vi "IMU.vi"(8 "error in (no error)":errorcluster, 10 "Acc/Gyro  address":u8, 11 "I2C Ref":T1) -> (3 "error out":errorcluster, 5 "IMU Acc":cluster{dbl, dbl, dbl}(graph), 6 "IMU Gyro":cluster{dbl, dbl, dbl}(graph))   [LabVIEW 2019]
uses:
  <vilib>/myRIO/Instrument Drivers/Onboard IO/I2C/typedefs/I2C Reference.ctl
  <vilib>/myRIO/Common/Instrument Driver Framework/Utilities/typedefs/myRIO Generic Hardware Reference.ctl
  <vilib>/myRIO/Common/Instrument Driver Framework/Utilities/typedefs/Hardware Version Enum.ctl
  <vilib>/myRIO/Common/Instrument Driver Framework/Utilities/typedefs/myRIO v1.0 Reference.ctl
  <vilib>/myRIO/Common/Instrument Driver Framework/Utilities/typedefs/Generic FPGA Reference.ctl
  <vilib>/myRIO/Common/Instrument Driver Framework/myRIO v1.0/I2C/typedefs/I2C Channels Enum.ctl
  <vilib>/myRIO/Instrument Drivers/Onboard IO/I2C/typedefs/I2C Configuration.ctl
  <vilib>/myRIO/Instrument Drivers/Onboard IO/I2C/typedefs/I2C Transfer Rate.ctl
  <vilib>/Utility/error.llb/Error Cluster From Error Code.vi
  <vilib>/myRIO/Common/Instrument Driver Framework/myRIO v1.0/I2C/vis/myRIO v1.0 Write I2C.vi
  <vilib>/myRIO/Common/Instrument Driver Framework/myRIO v1.0/I2C/vis/myRIO v1.0 Read I2C.vi
  <vilib>/myRIO/Instrument Drivers/Onboard IO/I2C/I2C.lvlib
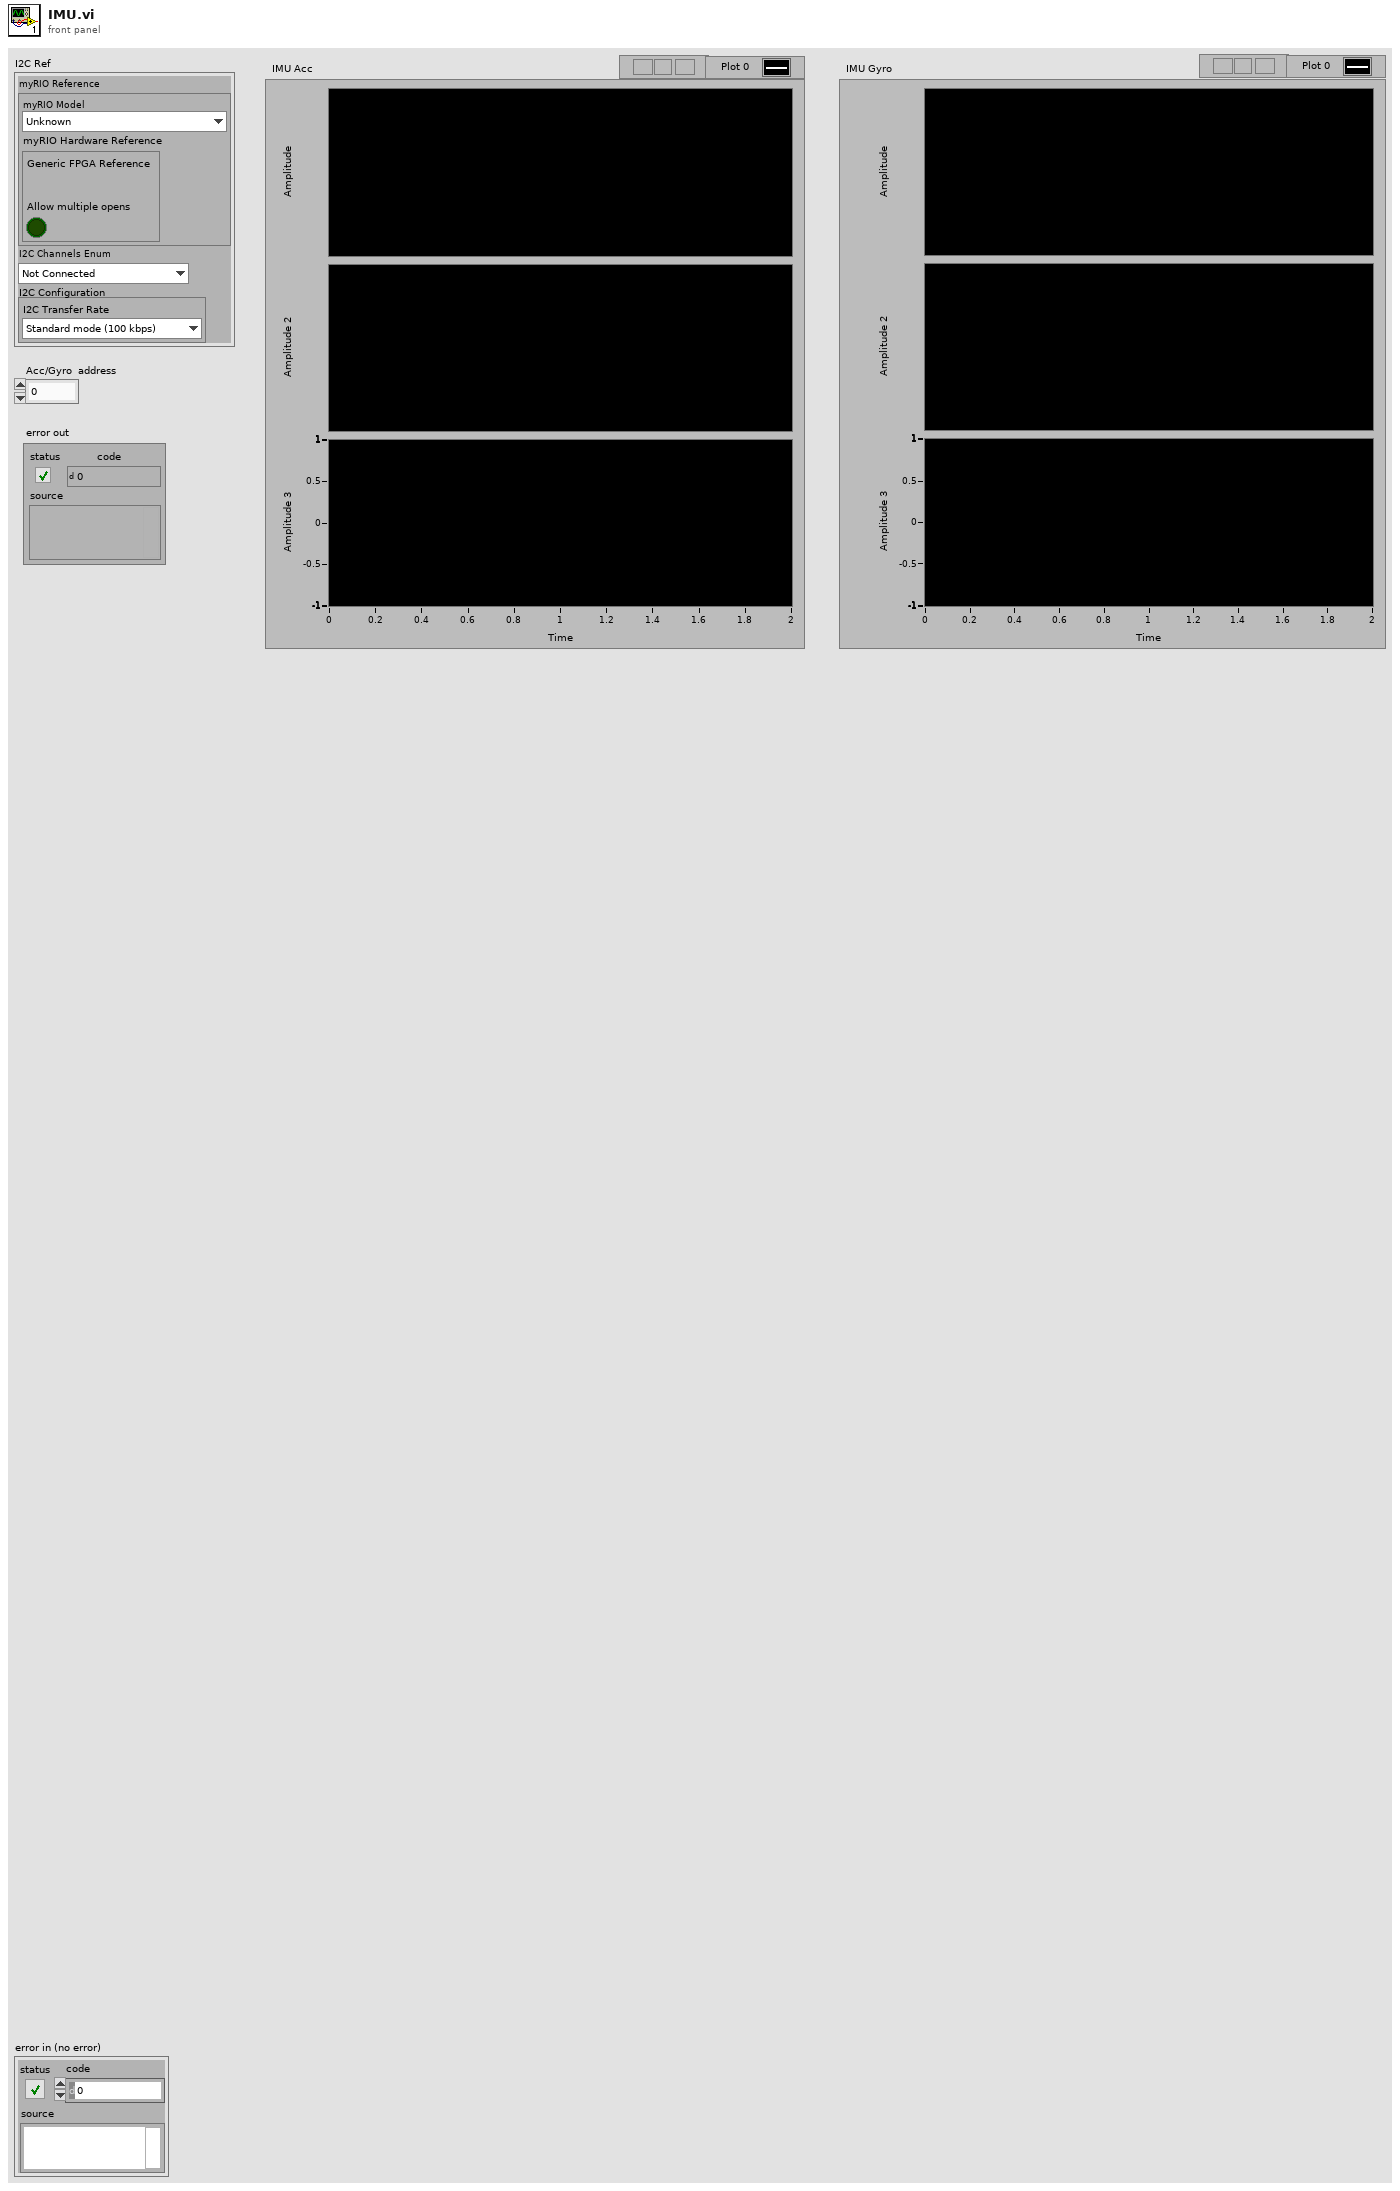
[diagram p1: front panel]
types:
  T1 = typedef "I2C.lvlib/I2C Reference.ctl" = cluster{"myRIO Reference":T2, "I2C Channels Enum":T6, "I2C Configuration":T7}
  T2 = typedef "myRIO Generic Hardware Reference.ctl" = cluster{"myRIO Model":T3, "myRIO Hardware Reference":T4}
  T3 = typedef "Hardware Version Enum.ctl" = enum16{"Unknown", "myRIO-1900", "myRIO-1950", "roboRIO", "NI ELVIS RIO CM", "ELVIS III"}
  T4 = typedef "myRIO v1.0 Reference.ctl" = cluster{"Generic FPGA Reference":T5, "Allow multiple opens":bool}
  T5 = typedef "Generic FPGA Reference.ctl" = refnum<k20>
  T6 = typedef "I2C Channels Enum.ctl" = enum16{"Not Connected", "A/I2C", "B/I2C", "I2C/I2C"}
  T7 = typedef "I2C.lvlib/I2C Configuration.ctl" = cluster{"I2C Transfer Rate":T8}
  T8 = typedef "I2C.lvlib/I2C Transfer Rate.ctl" = enum16{"Standard mode (100 kbps)", "Fast mode (400 kbps)"}
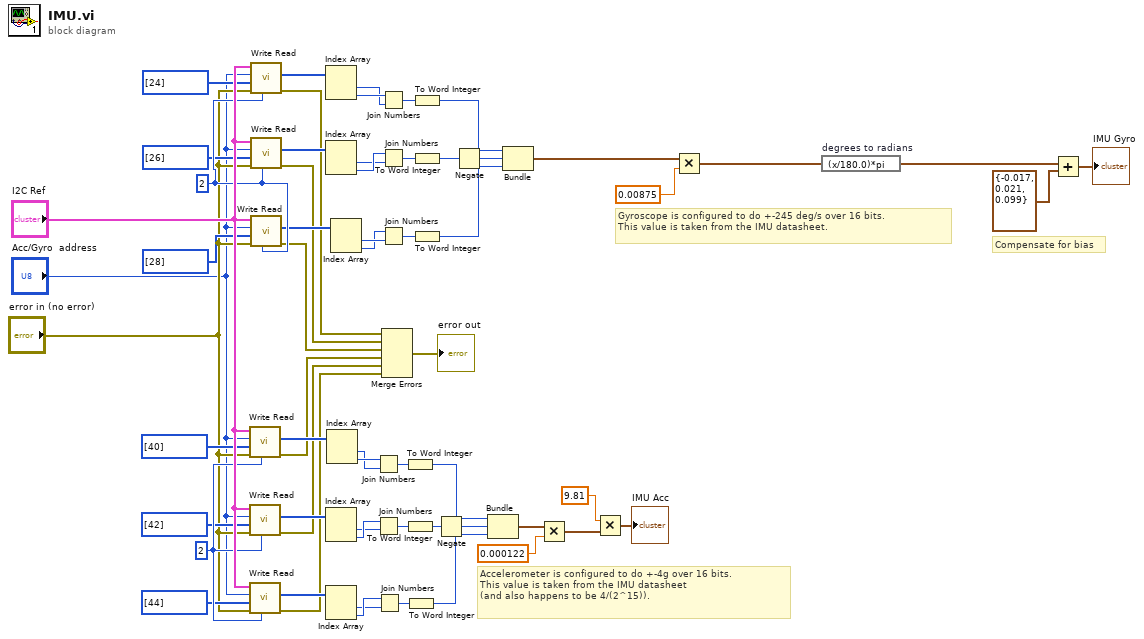
[diagram p0: block diagram]
diagram:
  w54 = u32 2 ("Byte Count")
  w40 = u32 2 ("Byte Count")
  # "Compensate for bias"
  # "Gyroscope is configured to do +-245 deg/s over 16 bits.\nThis value is taken from the IMU datasheet."
  # "Accelerometer is configured to do +-4g over 16 bits.\nThis value is taken from the IMU datasheet\n(and also happens to be 4/(2^15))."
  n1 = call <vilib>:"Write Read.vi"("Byte Count"=w40, "error in (no error)"="error in (no error)", "Bytes to Write"=u8[] [40], "Slave Address (7-bit)"="Acc/Gyro  address", "I2C Ref In"="I2C Ref") -> ("error out"=w19:errorcluster, "Bytes Read"=w32:u8[])  [unwired: 3 in, 1 out]
  n2 = call <vilib>:"Write Read.vi"("Byte Count"=w40, "error in (no error)"="error in (no error)", "Bytes to Write"=u8[] [42], "Slave Address (7-bit)"="Acc/Gyro  address", "I2C Ref In"="I2C Ref") -> ("error out"=w18:errorcluster, "Bytes Read"=w30:u8[])  [unwired: 3 in, 1 out]
  n3 = call <vilib>:"Write Read.vi"("Byte Count"=w40, "error in (no error)"="error in (no error)", "Bytes to Write"=u8[] [44], "Slave Address (7-bit)"="Acc/Gyro  address", "I2C Ref In"="I2C Ref") -> ("error out"=w17:errorcluster, "Bytes Read"=w28:u8[])  [unwired: 3 in, 1 out]
  n4 = call <vilib>:"Write Read.vi"("Byte Count"=w54, "error in (no error)"="error in (no error)", "Bytes to Write"=u8[] [24], "Slave Address (7-bit)"="Acc/Gyro  address", "I2C Ref In"="I2C Ref") -> ("error out"=w22:errorcluster, "Bytes Read"=w48:u8[])  [unwired: 3 in, 1 out]
  n5 = call <vilib>:"Write Read.vi"("Byte Count"=w54, "error in (no error)"="error in (no error)", "Bytes to Write"=u8[] [26], "Slave Address (7-bit)"="Acc/Gyro  address", "I2C Ref In"="I2C Ref") -> ("error out"=w21:errorcluster, "Bytes Read"=w46:u8[])  [unwired: 3 in, 1 out]
  n6 = call <vilib>:"Write Read.vi"("Byte Count"=w54, "error in (no error)"="error in (no error)", "Bytes to Write"=u8[] [28], "Slave Address (7-bit)"="Acc/Gyro  address", "I2C Ref In"="I2C Ref") -> ("error out"=w20:errorcluster, "Bytes Read"=w44:u8[])  [unwired: 3 in, 1 out]
  n7 = Index Array "Index Array"(array=w48) -> (element #1=w50:u8, element #2=w51:u8)  [unwired: 2 in]
  n8 = Index Array "Index Array"(array=w46) -> (element #1=w52:u8, element #2=w53:u8)  [unwired: 2 in]
  n9 = Index Array "Index Array"(array=w30) -> (element #1=w36:u8, element #2=w37:u8)  [unwired: 2 in]
  n10 = Index Array "Index Array"(array=w28) -> (element #1=w38:u8, element #2=w39:u8)  [unwired: 2 in]
  n11 = Index Array "Index Array"(array=w32) -> (element #1=w34:u8, element #2=w35:u8)  [unwired: 2 in]
  n12 = Index Array "Index Array"(array=w44) -> (element #1=w15:u8, element #2=w14:u8)  [unwired: 2 in]
  n13 = Join Numbers(hi=w35, lo=w34) -> ((hi.lo)=w25:u16)
  n14 = Join Numbers(hi=w37, lo=w36) -> ((hi.lo)=w26:u16)
  n15 = Join Numbers(hi=w39, lo=w38) -> ((hi.lo)=w27:u16)
  n16 = Join Numbers(hi=w51, lo=w50) -> ((hi.lo)=w41:u16)
  n17 = Join Numbers(hi=w53, lo=w52) -> ((hi.lo)=w42:u16)
  n18 = Join Numbers(hi=w14, lo=w15) -> ((hi.lo)=w43:u16)
  n19 = Merge Errors(w22, w21, w20, w19, w18, w17) -> (→"error out":errorcluster)
  n20 = To Word Integer(number=w25) -> (16bit integer=w60:i16)
  n21 = To Word Integer(number=w26) -> (16bit integer=w59:i16)
  n22 = To Word Integer(number=w27) -> (16bit integer=w58:i16)
  n23 = To Word Integer(number=w41) -> (16bit integer=w13:i16)
  n24 = To Word Integer(number=w42) -> (16bit integer=w8:i16)
  n25 = To Word Integer(number=w43) -> (16bit integer=w12:i16)
  n26 = Negate(x=w59) -> (-x=w9:i16)
  n27 = Negate(x=w8) -> (-x=w7:i16)
  n28 = Bundle "Bundle"(w60, w9, w58) -> (w56:cluster{i16, i16, i16})  [unwired: 1 in]
  n29 = Bundle "Bundle"(w13, w7, w12) -> (w6:cluster{i16, i16, i16})  [unwired: 1 in]
  n30 = Multiply(x=w56, y=0.000122) -> (x*y=w57:cluster{dbl, dbl, dbl})
  n31 = Multiply(x=9.81 ("y"), y=w57) -> (x*y=→"IMU Acc":cluster{dbl, dbl, dbl})
  n32 = Multiply(x=w6, y=0.00875) -> (x*y=w2:cluster{dbl, dbl, dbl})
  n33 = expression code="(x/180.0)*pi" "degrees to radians"(w2) -> (w3:cluster{dbl, dbl, dbl})
  n34 = Add(x=w3, y=cluster{dbl, dbl, dbl} {-0.017, 0.021, 0.099}) -> (x+y=→"IMU Gyro":cluster{dbl, dbl, dbl})
